vi "GlobalV.vi"() -> ()   [LabVIEW 2013]
panel:
  in  "Stop":bool
  in  "SelfMode":string[](array[string])
  in  "BSJMode":string[](array[string])
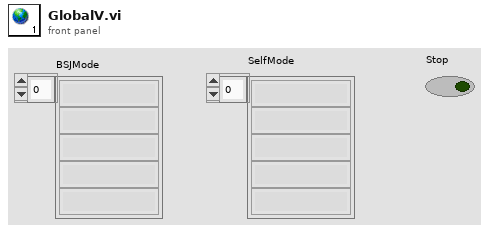
[diagram p1: front panel]
diagram:
